vi "Read Example With Events (advanced).vi"() -> ()   [LabVIEW 2016]
uses:
  type defs/Data In.ctl
  library/GEA2_Toolkit.lvlib
panel:
  out "Count":dbl
  out "x = y?":bool
  out "Message":string=" 00 00 01 0C 64 1E 40 0A 04 10 00 10 02 00 02 00 00 00 41 00 EF 03 94 6C 00 00"
  out "Error Out":errorcluster
  in  "Send":bool
  in  "Input Data":T1={"Source"=228, "Destination"=37, "Command"=158, "Message"=""} {"Command" format="%02x"; "Destination" format="%02x"; "Source" format="%02x"}
  in  "Stop":bool
  out "Log":string="10/16/15 13:13:24.219 RECV 19 E4 50 00 00 00 00 00 02\r\n10/16/15 13:13:24.345 RECV 19 E4 41 01 00 00 00 00 00 00 00 00 00 00 00 00 00 00 00 07 6C 00 8F 11 20 00 00 00 49\r\n10/16/15 13:13:24.410 RECV 19 E4 60 54 54 00 00 03 31 33 00 00 00 00 35 FF FF FF FF 00 00 00 00 01\r\n10/16/15 13:13:25.217 RECV 19 E4 50 00 00 00 00 00 02\r\n10/16/15 13:13:25.345 RECV 19 E4 41 01 00 00 00 00 00 00 00 00 00 00 00 00 00 00 00 07 6C 00 8F 11 20 00 00 00 49\r\n10/16/15 13:13:25.409 RECV 19 E4 60 54 54 00 00 03 31 33 00 00 00 00 35 FF FF FF FF 00 00 00 00 01\r\n10/16/15 13:13:26.215 RECV 19 E4 50 00 00 00 00 00 02\r\n10/16/15 13:13:26.379 RECV 19 E4 41 01 00 00 00 00 00 00 00 00 00 00 00 00 00 00 00 07 6C 00 8F 11 20 00 00 00 49\r\n10/16/15 13:13:26.494 RECV 19 E4 60 54 54 00 00 03 31 33 00 00 00 00 35 FF FF FF FF 00 00 00 00 01\r\n10/16/15 13:13:26.698 RECV 19 E4 40 00 00 00 00 21 02 01 01\r\n10/16/15 13:13:27.021 RECV 19 E4 9E 00 00 01 0C 64 1E 40 0A 04 10 00 10 02 00 02 00 00 00 41 00 EF 03 94 6C 00 00\r\n10/16/15 13:13:27.215 RECV 19 E4 50 00 00 00 00 00 02\r\n10/16/15 13:13:27.340 RECV 19 E4 41 01 00 00 00 00 00 00 00 00 00 00 00 00 00 00 00 07 6C 00 8F 11 20 00 00 00 49\r\n10/16/15 13:13:27.404 RECV 19 E4 60 54 54 00 00 03 31 33 00 00 00 00 35 FF FF FF FF 00 00 00 00 01\r\n10/16/15 13:13:28.211 RECV 19 E4 50 00 00 00 00 00 02\r\n10/16/15 13:13:28.338 RECV 19 E4 41 01 00 00 00 00 00 00 00 00 00 00 00 00 00 00 00 07 6C 00 8F 11 20 00 00 00 49\r\n10/16/15 13:13:28.403 RECV 19 E4 60 54 54 00 00 03 31 33 00 00 00 00 35 FF FF FF FF 00 00 00 00 01\r\n10/16/15 13:13:29.211 RECV 19 E4 50 00 00 00 00 00 02\r\n10/16/15 13:13:29.338 RECV 19 E4 41 01 00 00 00 00 00 00 00 00 00 00 00 00 00 00 00 07 6C 00 8F 11 20 00 00 00 49\r\n10/16/15 13:13:29.386 RECV 19 E4 74 72 72 45 76 6E 49 0A 0D 42 45 2D 30 30 30 30 3A 30 62 72 72 45 76 6E 49 0A 0D 41 45 2D\r\n10/16/15 13:13:29.415 RECV 19 E4 50 00 00 00 00 00 02\r\n10/16/15 13:13:29.452 RECV 19 E4 60 54 54 00 00 03 31 33 00 00 00 00 35 FF FF FF FF 00 00 00 00 02\r\n10/16/15 13:13:29.492 RECV 19 E4 74 0D 44 45 2D 30 30 30 30 3A 32 62 72 72 45 76 6E 49 0A 0D 43 45 2D 30 30 30 30 3A 31 62\r\n10/16/15 13:13:29.520 RECV 19 E4 50 01 00 00 00 01 02\r\n10/16/15 13:13:29.566 RECV 19 E4 74 30 30 30 5B 73 74 6C 75 61 46 0A 0D 45 45 2D 30 30 30 30 3A 33 62 72 72 45 76 6E 49 0A\r\n10/16/15 13:13:29.604 RECV 19 E4 74 30 0A 0D 31 46 2D 2C 39 31 32 30 0A 0D 30 46 2D 2C 39 32 32 30 0A 0D 46 45 2D 3A 5D 38\r\n10/16/15 13:13:29.644 RECV 19 E4 74 0A 0D 34 46 2D 2C 30 31 32 30 0A 0D 33 46 2D 2C 32 31 32 30 0A 0D 32 46 2D 2C 37 30 32\r\n10/16/15 13:13:29.682 RECV 19 E4 74 0D 37 46 2D 2C 33 31 30 30 0A 0D 36 46 2D 2C 38 31 30 30 0A 0D 35 46 2D 2C 32 30 31 30\r\n10/16/15 13:13:29.723 RECV 19 E4 74 6B 61 72 42 20 3A 43 49 0A 0D 38 46 2D 4D 53 46 20 6E 69 70 53 20 40 20 65 6C 64 49 0A\r\n10/16/15 13:13:29.767 RECV 19 E4 74 70 53 20 40 20 79 72 74 6E 45 0A 0D 39 46 2D 30 30 30 30 20 30 30 30 30 20 57 43 20 65\r\n10/16/15 13:13:29.809 RECV 19 E4 74 30 30 30 30 20 44 4E 55 20 3A 53 49 0A 0D 41 46 2D 65 76 69 74 69 6D 69 72 50 20 6E 69\r\n10/16/15 13:13:29.865 RECV 19 E4 74 75 52 0A 0D 42 46 2D 35 33 30 30 20 31 30 30 30 2D 20 31 30 30 30 2D 20 30 30 30 30 20\r\n10/16/15 13:13:29.910 RECV 19 E4 74 43 43 20 65 6B 61 72 42 20 3A 43 49 0A 0D 43 46 2D 4D 53 46 20 6E 69 70 53 20 40 20 6E\r\n10/16/15 13:13:30.009 RECV 19 E4 74 46 46 46 46 20 30 30 30 30 20 3A 44 4C 0A 0D 44 46 2D 31 30 30 30 20 30 30 30 30 20 57\r\n10/16/15 13:13:30.078 RECV 19 E4 74 31 30 30 20 46 46 4F 20 4F 20 4F 20 46 46 4F 20 54 45 53 20 55 20 4F 4C 20 32 30 33 43\r\n10/16/15 13:13:30.118 RECV 19 E4 9E 00 00 01 0C 64 1E 40 0A 04 10 00 10 02 00 02 00 00 00 41 00 EF 03 94 6C 00 00\r\n10/16/15 13:13:30.194 RECV 19 E4 74 20 55 20 4F 4C 20 32 30 33 43 46 46 46 46 20 30 32 30 30 20 3A 44 4C 0A 0D 45 46 2D 35\r\n10/16/15 13:13:30.217 RECV 19 E4 50 01 00 00 00 01 02\r\n10/16/15 13:13:30.281 RECV 19 E4 74 35 31 30 30 20 46 46 4F 20 4F 20 4F 20 46 46 4F 20 54 45 53\r\n10/16/15 13:13:30.354 RECV 19 E4 41 01 00 00 00 00 00 00 00 00 00 00 00 00 00 00 00 07 6C 00 8F 11 20 00 00 00 49\r\n10/16/15 13:13:30.421 RECV 19 E4 60 54 54 00 00 03 31 33 00 00 00 00 35 FF FF FF FF 00 00 00 00 02\r\n10/16/15 13:13:31.209 RECV 19 E4 50 01 00 00 00 01 02\r\n10/16/15 13:13:31.334 RECV 19 E4 41 01 00 00 00 00 00 00 00 00 00 00 00 00 00 00 00 07 6C 00 8F 11 20 00 00 00 49\r\n10/16/15 13:13:31.399 RECV 19 E4 60 54 54 00 00 03 31 33 00 00 00 00 35 FF FF FF FF 00 00 00 00 02\r\n10/16/15 13:13:31.762 RECV 19 E4 40 00 00 00 00 21 02 01 01\r\n10/16/15 13:13:32.218 RECV 19 E4 50 01 00 00 00 01 02\r\n10/16/15 13:13:32.254 RECV 19 E4 9E 00 00 01 0C 64 1E 40 0A 04 10 00 10 02 00 02 00 00 00 41 00 EF 03 94 6C 00 00\r\n10/16/15 13:13:32.333 RECV 19 E4 41 01 00 00 00 00 00 00 00 00 00 00 00 00 00 00 00 07 6C 00 8F 11 20 00 00 00 49\r\n10/16/15 13:13:32.399 RECV 19 E4 60 54 54 00 00 03 31 33 00 00 00 00 35 FF FF FF FF 00 00 00 00 02\r\n10/16/15 13:13:33.205 RECV 19 E4 50 01 00 00 00 01 02\r\n10/16/15 13:13:33.331 RECV 19 E4 41 01 00 00 00 00 00 00 00 00 00 00 00 00 00 00 00 07 6C 00 8F 11 20 00 00 00 49\r\n10/16/15 13:13:33.424 RECV 19 E4 60 54 54 00 00 03 31 33 00 00 00 00 35 FF FF FF FF 00 00 00 00 02\r\n10/16/15 13:13:34.204 RECV 19 E4 50 01 00 00 00 01 02\r\n10/16/15 13:13:34.329 RECV 19 E4 41 01 00 00 00 00 00 00 00 00 00 00 00 00 00 00 00 07 6C 00 8F 11 20 00 00 00 49\r\n10/16/15 13:13:34.394 RECV 19 E4 60 54 54 00 00 03 31 33 00 00 00 00 35 FF FF FF FF 00 00 00 00 02\r\n10/16/15 13:13:35.203 RECV 19 E4 50 01 00 00 00 01 02\r\n10/16/15 13:13:35.329 RECV 19 E4 41 01 00 00 00 00 00 00 00 00 00 00 00 00 00 00 00 07 6C 00 8F 11 20 00 00 00 49\r\n"
  in  "Error In":errorcluster
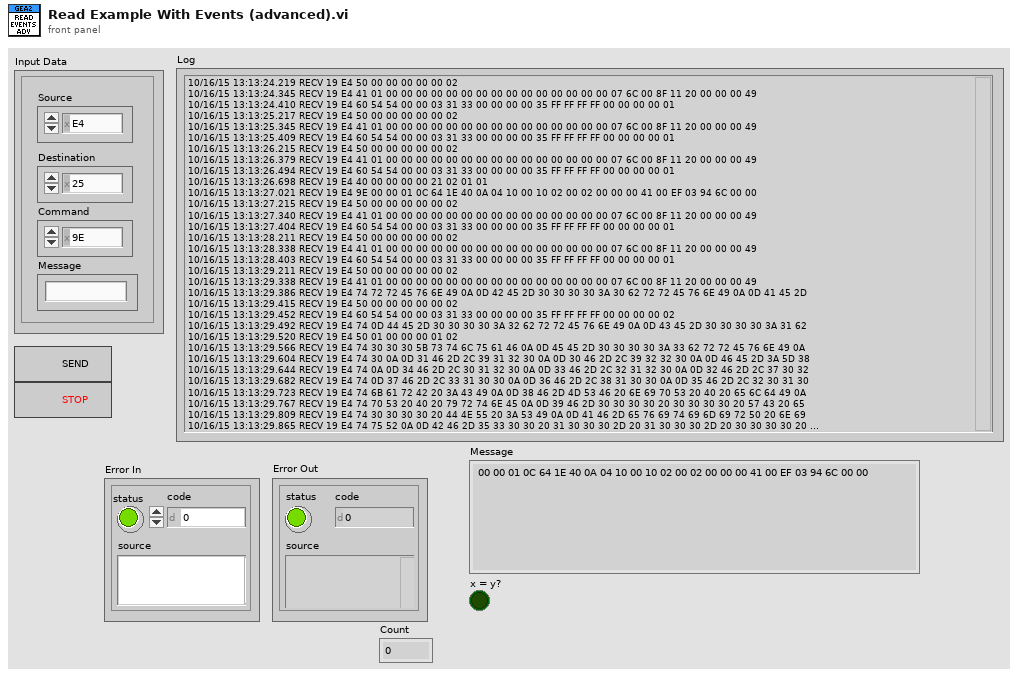
[diagram p1: front panel]
types:
  T1 = typedef "GEA2_Toolkit.lvlib/Data In.ctl" = cluster{"Source":u8, "Destination":u8, "Command":u8, "Message":string}
  T2 = typedef "eventsource.ctl" = u32
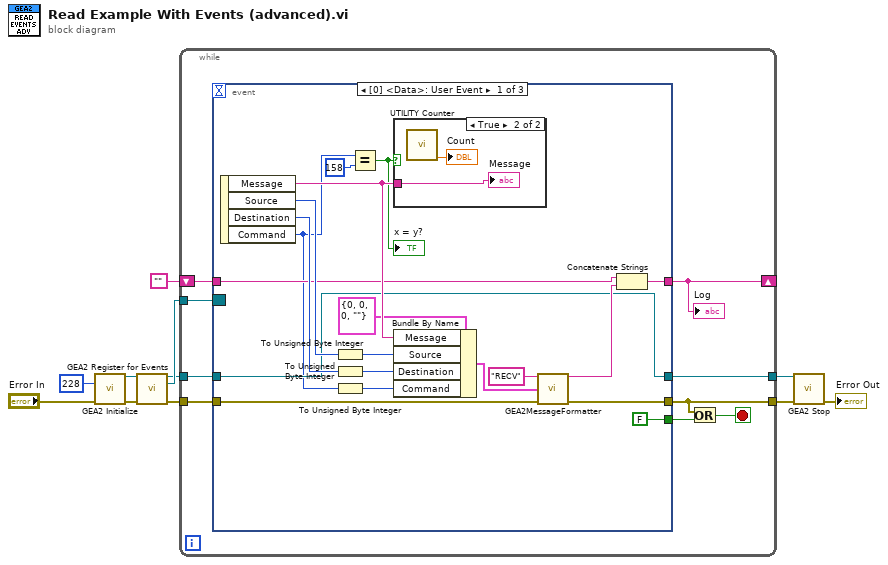
[diagram p0: block diagram]
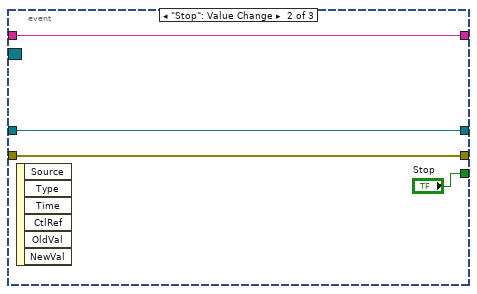
[diagram p3: hidden frame]
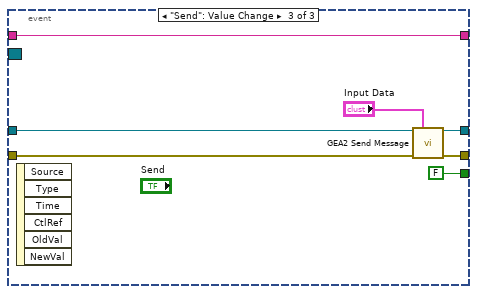
[diagram p4: hidden frame]
diagram:
  n1 = call "GEA2 Initialize.vi"("Source Address"=u8 228, "error in"="Error In") -> ("GEA2 Reference Out"=w10:refnum<k24>, "error out"=w11:errorcluster)  [unwired: 11 in, 1 out]
  n2 = call "GEA2 Register for Events.vi"("GEA2 Reference In"=w10, "Error In"=w11) -> ("GEA2 Reference Out"=w4:refnum<k24>, "GEA2 Event Registration"=w7:refnum<event-registration>, "Error Out"=w6:errorcluster)  [unwired: 11 in]
  n3 = while {
    tunnel: w7 -> [w20]
    tunnel: w6 -> [w19]
    shift-right: [w17] -> _
    shift-left: "" -> [w18]
    tunnel: w4 -> [w16]
    tunnel: [w15] -> w3
    tunnel: [w14] -> w2
    stop <- w12 stop-if-true
    n4 = event shown="[0] <Data>: User Event" {
      selector: w20 -> [_ _ _]
      dyn-events: _ -> [_ _ _]
      timeout: _ -> [_ _ _]
      tunnel: w19 -> [w30 w44 w50]
      tunnel: [w29 w44 w49] -> w14
      tunnel: w18 -> [w28 w43 w52]
      tunnel: [w26 w43 w52] -> w17
      tunnel: w16 -> [w25 w42 w48]
      tunnel: [w25 w42 w47] -> w15
      tunnel: [FALSE "Stop" FALSE ("Stop")] -> w13
      event User Event {
        n5 = event-data() -> ("Message"=w34:string, "Source"=w35:T2, "Destination"=w36:u8, "Command"=w23:u8)  [unwired: 1 in]
        n6 = To Unsigned Byte Integer(number=w35) -> (unsigned 8bit integer=w38:u8)
        n7 = To Unsigned Byte Integer(number=w36) -> (unsigned 8bit integer=w39:u8)
        n8 = To Unsigned Byte Integer(number=w23) -> (unsigned 8bit integer=w37:u8)
        n9 = Equal?(x=w23, y=u8 158) -> (x = y?=w21:bool)
        "x = y?" <- w21
        n10 = case shown="True" w21 {
          tunnel: w34 -> [_ w41]
          frame False {
          }
          frame True {
            n11 = call "UTILITY Counter.vi"() -> ("Count"=→"Count":dbl)  [unwired: 11 in]
            "Message" <- w41
          }
        }
        n12 = Bundle By Name(cluster=T1 {"Source"=0, "Destination"=0, "Command"=0, "Message"=""} ("Data In"), "Message"=w34, "Source"=w38, "Destination"=w39, "Command"=w37) -> (w32:T1)
        n13 = call "GEA2MessageFormatter.vi"("Prefix(Send/Recv)"="RECV", "GEA2 Data In"=w32, "Error In"=w30) -> ("Output String"=w27:string, "Error Out"=w29:errorcluster)  [unwired: 11 in]
        n14 = Concatenate Strings(w28, w27) -> (w26:string)
      }
      event "Stop": Value Change {
        n15 = event-data() -> ()  [unwired: 1 in, 6 out]
      }
      event "Send": Value Change {
        n16 = event-data() -> ()  [unwired: 1 in, 6 out]
        n17 = call "GEA2 Send Message.vi"("GEA2 Reference In"=w48, "Input Data"="Input Data", "Error In"=w50) -> ("GEA2 Reference Out"=w47:refnum<k24>, "Error Out"=w49:errorcluster)  [unwired: 11 in]
      }
    }
    "Log" <- w17
    n18 = Or(x=w14, y=w13) -> (x .or. y?=w12:bool)
  }
  n19 = call "GEA2 Stop.vi"("GEA2 Reference Out"=w3, "Error In"=w2) -> ("Error Out"=→"Error Out":errorcluster)  [unwired: 13 in]
